vi "checkTempTransitionTimeElapsed.vi"(8 "error in (no error)":errorcluster, 11 "Model in":refnum<class "Model.lvclass">) -> (0 "error out":errorcluster, 2 "tempTransitionTimeHasElapsedIsTrue":bool, 3 "Model out":refnum<class "Model.lvclass">)   [LabVIEW 2013, in "Model.lvclass"]
uses:
  Model.lvclass
  Model.lvclass/Model.ctl
  UserEvents/UserEvents.lvclass/UserEvents.ctl
  ApplicationElements/TestMonitor/TestMonitor.lvclass
  UserEvents/UserEvents.lvclass
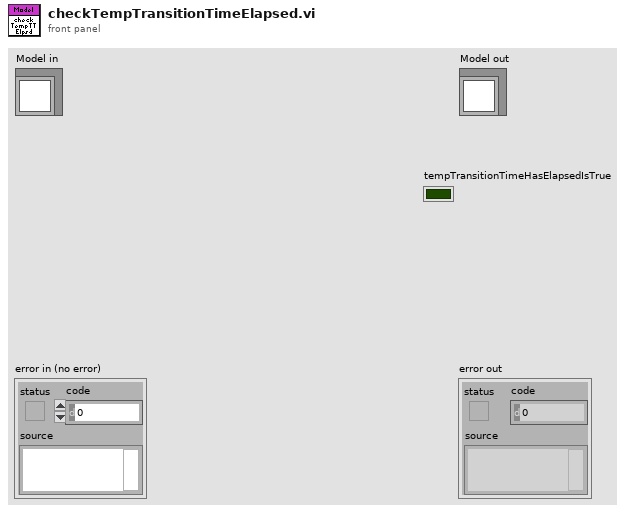
[diagram p1: front panel]
types:
  T1 = typedef "AITDTTypedefs.lvlib/PubDataEvents.ctl" = cluster{"State":refnum<user-event>, "ErrorCode":refnum<user-event>, "OutputData":refnum<user-event>, "InputData":refnum<user-event>, "TestStatus":refnum<user-event>, "LogPath":refnum<user-event>, "TemperatureSetpointRequest":refnum<user-event>, "TemperatureSettling":refnum<user-event>, "WaitTimeStatus":refnum<user-event>}
  T2 = typedef "AITDTTypedefs.lvlib/WaitTimeStatus.ctl" = cluster{"Time Remaining":dbl[unit]}
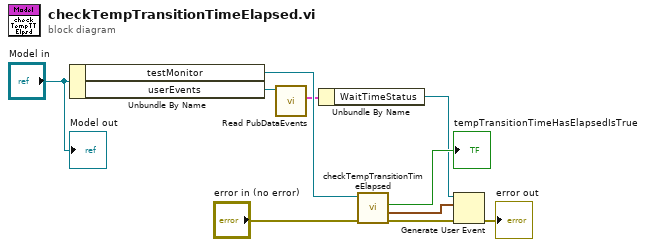
[diagram p0: block diagram]
diagram:
  n1 = Unbundle By Name("Model in") -> ("testMonitor"=w9:refnum<class "TestMonitor.lvclass">, "userEvents"=w6:refnum<class "UserEvents.lvclass">)
  n2 = call "Read PubDataEvents.vi"("UserEvents in"=w6) -> ("PubDataEvents"=w7:T1)  [unwired: 9 in, 1 out]
  n3 = Unbundle By Name(w7) -> ("WaitTimeStatus"=w2:refnum<user-event>)
  n4 = call "checkTempTransitionTimeElapsed.vi"("error in (no error)"="error in (no error)", "TestMonitor in"=w9) -> ("error out"=w4:errorcluster, "Wait Time Status"=w5:T2, "tempTransitionTimeElapsedIsTrue"=→"tempTransitionTimeHasElapsedIsTrue":bool)  [unwired: 6 in, 1 out]
  n5 = Generate User Event(user event=w2, event data cluster=w5, error in=w4) -> (error out=→"error out":errorcluster)  [unwired: 1 in, 1 out]
  "Model out" <- "Model in"
